vi "Launcher.vi"() -> ()   [LabVIEW 2024]
uses:
  UIType.ctl
  UserLevel.ctl
  UI Manager Proxy_class/UI Manager Proxy.lvclass
  <vilib>/Utility/miscctls.llb/LVRectTypeDef.ctl
panel:
  in  "User Level":T1
  in  "ChangeUserLevel":bool
  in  "UI Type":T2=enum."Debugging Page"
  in  "OpenNewPage":bool
  # "398 × 286"
  # "Made by Ramazan Burak Korkmaz"
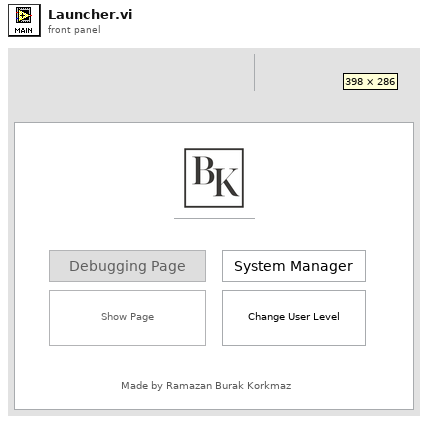
[diagram p1: front panel]
types:
  T1 = typedef "UserLevel.ctl" = enum16{"System Manager", "Admin", "Operator"}
  T2 = typedef "UIType.ctl" = enum16{"Main Page", "Settings Page", "Debugging Page"}
  T3 = enum8{"Enabled", "Disabled", "Disabled and Grayed Out"}
  T4 = typedef "LVRectTypeDef.ctl" = cluster{"Left":i16, "Top":i16, "Right":i16, "Bottom":i16}
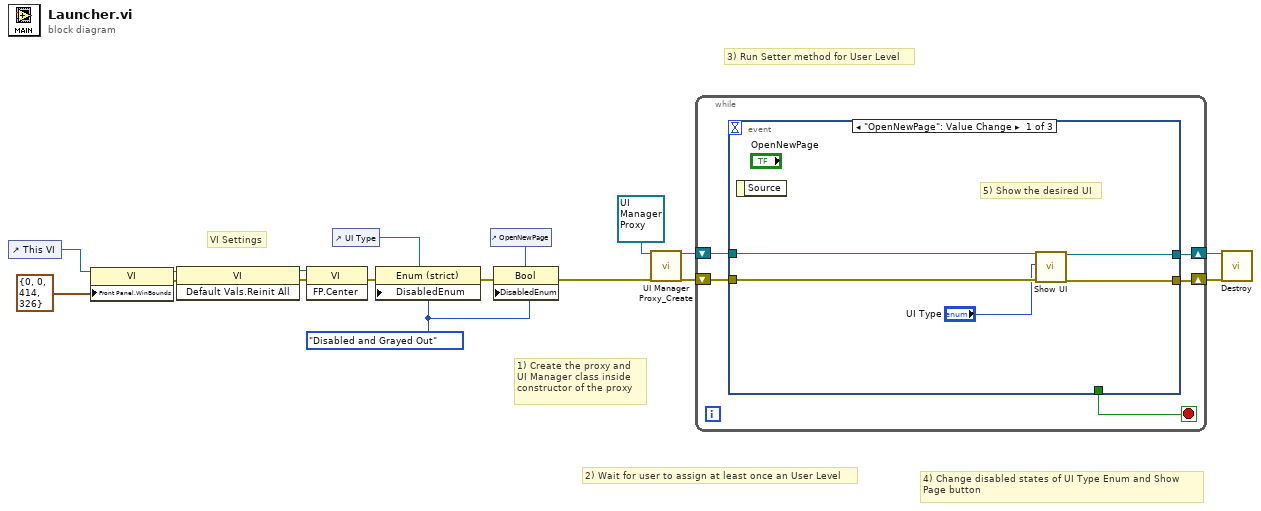
[diagram p0: block diagram]
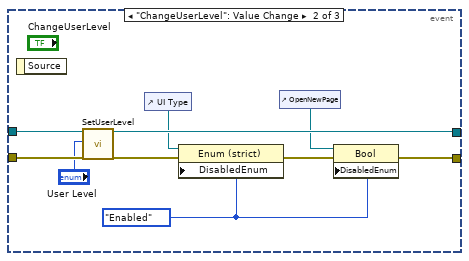
[diagram p2: hidden frame]
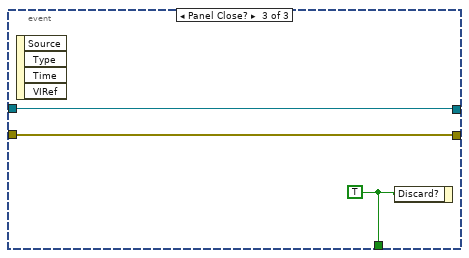
[diagram p3: hidden frame]
diagram:
  w1 = T3."Disabled and Grayed Out" ("Disabled")
  # "VI Settings"
  # "4) Change disabled states of UI Type Enum and Show\nPage button"
  # "3) Run Setter method for User Level"
  # "2) Wait for user to assign at least once an User Level"
  # "1) Create the proxy and\nUI Manager class inside\nconstructor of the proxy"
  n1 = control-ref of="This VI"() -> (w7:refnum<vi>)
  n2 = property class="VI"(reference=w7, "Front Panel.WinBounds"=T4 {"Left"=0, "Top"=0, "Right"=414, "Bottom"=326} ("Front Panel Window:Window Bounds")) -> (reference out=w8:refnum<vi>, error out=w9:errorcluster)  [unwired: 1 in]
  n3 = invoke class="VI" method="Default Vals.Reinit All"(reference=w8, error in=w9) -> (reference out=w10:refnum<vi>, error out=w11:errorcluster)  [unwired: 1 in, 1 out]
  n4 = invoke class="VI" method="FP.Center"(reference=w10, error in=w11) -> (error out=w6:errorcluster)  [unwired: 1 in, 2 out]
  n5 = control-ref of="UI Type"() -> (w4:refnum<vi>)
  n6 = property class="Enum (strict)"(reference=w4, error in=w6, "DisabledEnum"=w1) -> (error out=w5:errorcluster)  [unwired: 1 out]
  n7 = control-ref of="OpenNewPage"() -> (w2:refnum<vi>)
  n8 = property class="Bool"(reference=w2, error in=w5, "DisabledEnum"=w1) -> (error out=w3:errorcluster)  [unwired: 1 out]
  n9 = call "UI Manager Proxy_Create.vi"("reference in"=refnum<class "UI Manager Proxy.lvclass"> refnum ("UI Manager Proxy"), "Error In"=w3) -> ("reference out"=w17:refnum<class "UI Manager Proxy.lvclass">, "Error Out"=w16:errorcluster)  [unwired: 16 in]
  n10 = while {
    shift-right: [w20] -> w14
    shift-left: w17 -> [w22]
    shift-right: [w19] -> w13
    shift-left: w16 -> [w21]
    stop <- w18 stop-if-true
    n11 = event shown="[0] \"OpenNewPage\": Value Change" {
      selector: _ -> [_ _ _]
      dyn-events: _ -> [_ _ _]
      timeout: _ -> [_ _ _]
      tunnel: w22 -> [w27 w35 w40]
      tunnel: w21 -> [w26 w37 w39]
      tunnel: [w24 w34 w40] -> w20
      tunnel: [w23 w30 w39] -> w19
      tunnel: [_ _ w38] -> w18
      event "OpenNewPage": Value Change {
        # "5) Show the desired UI"
        n12 = event-data() -> ()  [unwired: 1 in, 1 out]
        n13 = call-dynamic "Show UI.vi"("reference in"=w27, "UI Type"="UI Type", "Error In"=w26) -> ("reference out"=w24:refnum<class "UI Manager Proxy.lvclass">, "Error Out"=w23:errorcluster)  [unwired: 15 in]
      }
      event "ChangeUserLevel": Value Change {
        w28 = T3."Enabled" ("Disabled")
        n14 = event-data() -> ()  [unwired: 1 in, 1 out]
        n15 = call-dynamic "SetUserLevel.vi"("reference in"=w35, "UserLevel"="User Level", "Error In"=w37) -> ("reference out"=w34:refnum<class "UI Manager Proxy.lvclass">, "Error Out"=w36:errorcluster)  [unwired: 15 in]
        n16 = control-ref of="UI Type"() -> (w31:refnum<vi>)
        n17 = property class="Enum (strict)"(reference=w31, error in=w36, "DisabledEnum"=w28) -> (error out=w32:errorcluster)  [unwired: 1 out]
        n18 = control-ref of="OpenNewPage"() -> (w29:refnum<vi>)
        n19 = property class="Bool"(reference=w29, error in=w32, "DisabledEnum"=w28) -> (error out=w30:errorcluster)  [unwired: 1 out]
      }
      event Panel Close? {
        w38 = TRUE ("Discard?")
        n20 = event-data() -> ()  [unwired: 1 in, 4 out]
        n21 = event-data("Discard?"=w38) -> ()  [unwired: 1 in, 1 out]
      }
    }
  }
  n22 = call-dynamic "Destroy.vi"("reference in"=w14, "Error In"=w13) -> ()  [unwired: 16 in, 2 out]
